vi "calculateWaveformTime.vi"(8 "error in (no error)":errorcluster, 11 "GuassianNoiseWave in":refnum<class "GuassianNoiseWave.lvclass">) -> (0 "error out":errorcluster, 2 "Waveform Time":dbl[unit], 3 "GuassianNoiseWave out":refnum<class "GuassianNoiseWave.lvclass">)   [LabVIEW 2015, in "GuassianNoiseWave.lvclass"]
uses:
  GuassianNoiseWave.lvclass
  GuassianNoiseWave.lvclass/GuassianNoiseWave.ctl
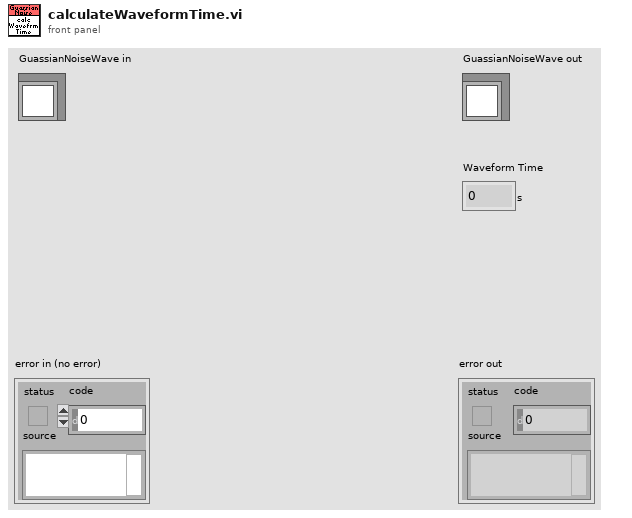
[diagram p1: front panel]
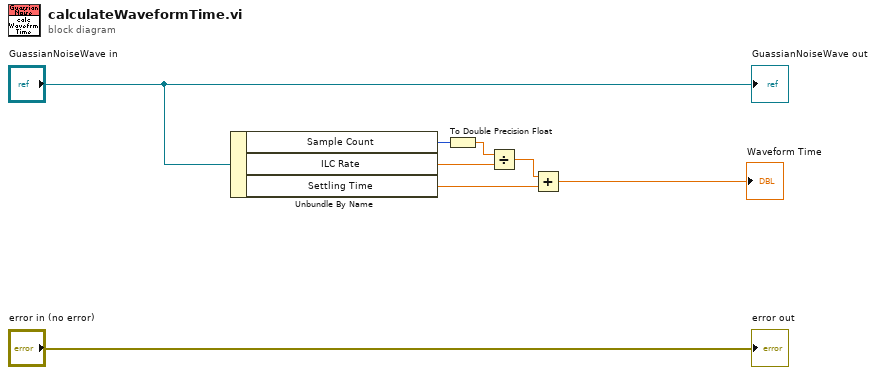
[diagram p0: block diagram]
diagram:
  n1 = Unbundle By Name("GuassianNoiseWave in") -> ("Sample Count"=w6:u32, "ILC Rate"=w5:dbl[unit], "Settling Time"=w3:dbl[unit])
  n2 = To Double Precision Float(number=w6) -> (double precision float=w7:dbl)
  n3 = Divide(x=w7, y=w5) -> (x/y=w4:dbl[unit])
  n4 = Add(x=w4, y=w3) -> (x+y=→"Waveform Time":dbl[unit])
  "error out" <- "error in (no error)"
  "GuassianNoiseWave out" <- "GuassianNoiseWave in"
